vi "Copy.vi"(11 "TypedCircularBuffer in":refnum<class "LogCircularBuffer.lvclass">) -> (2 "Copied Buffer":T1[](array[typedef]), 3 "TypedCircularBuffer out":refnum<class "LogCircularBuffer.lvclass">)   [LabVIEW 2024, in "LogCircularBuffer.lvclass"]
uses:
  LogCircularBuffer.lvclass
  Type.ctl
  RQMHCore/ErrorReporting/Record/LogRecord.lvclass
  LogCircularBuffer.lvclass/LogCircularBuffer.ctl
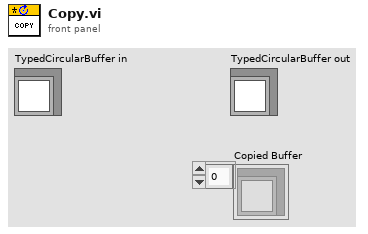
[diagram p1: front panel]
types:
  T1 = typedef "LogCircularBuffer.lvclass/Type.ctl" = refnum<class "LogRecord.lvclass">
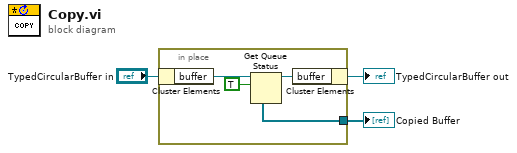
[diagram p0: block diagram]
diagram:
  n1 = in-place {
    in-place-border: [w4] -> w1
    n2 = in-place-cluster #1("TypedCircularBuffer in") -> ("buffer"=w7:refnum<queue>)
    n3 = Get Queue Status(queue=w7, return elements? (F)=TRUE) -> (queue out=w6:refnum<queue>, elements=w4:T1[])  [unwired: 1 in, 6 out]
    n4 = in-place-cluster #1("buffer"=w6) -> (→"TypedCircularBuffer out":refnum<class "LogCircularBuffer.lvclass">)
  }
  "Copied Buffer" <- w1
